vi "Save File Parse File Name RLT.vi"(8 "Error In":errorcluster, 11 "File String Name":path=path "C:/Users/220038920/Desktop/TR_S21_Lab ID_S21_SN_S21_Cycle_0_ClothWeight_8.45lbs_DOE_Exhaust_AHAM_20170703_File0_Inv and MC.csv") -> (0 "Error Out":errorcluster, 1 "Serial Number":string, 2 "Cycle":string, 3 "Date":string, 4 "Lab ID":string, 6 "TR Number":string)   [LabVIEW 2016, in "Save File.lvlib"]
uses:
  Save File.lvlib
  <vilib>/Utility/error.llb/whitespace.ctl
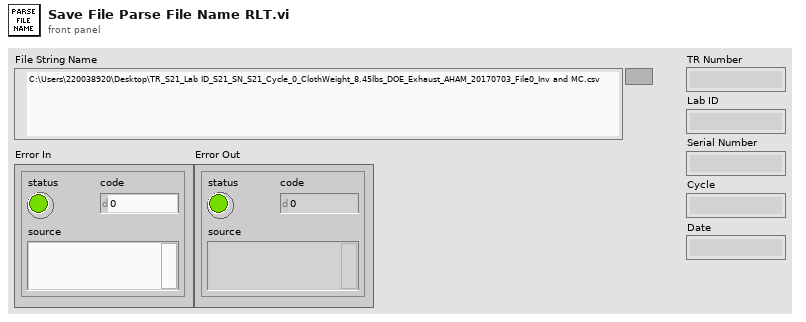
[diagram p1: front panel]
types:
  T1 = typedef "whitespace.ctl" = u16
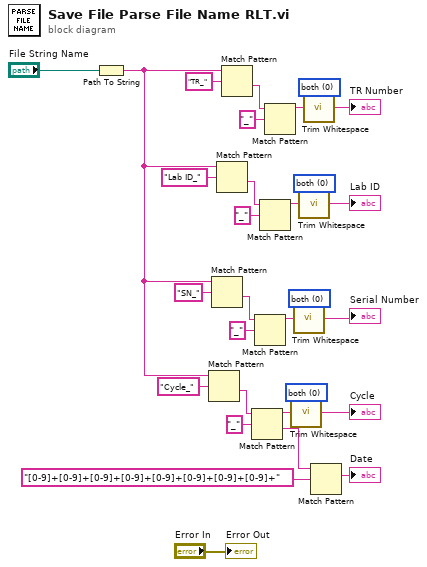
[diagram p0: block diagram]
diagram:
  w12 = T1 0 items=["both", "start of string", "end of string"] ("location (both)")
  w13 = T1 0 items=["both", "start of string", "end of string"] ("location (both)")
  w22 = T1 0 items=["both", "start of string", "end of string"] ("location (both)")
  w23 = T1 0 items=["both", "start of string", "end of string"] ("location (both)")
  n1 = Path To String(path="File String Name") -> (string=w4:string)
  n2 = Match Pattern(string=w4, regular expression="Cycle_") -> (after substring=w9:string)  [unwired: 1 in, 3 out]
  n3 = Match Pattern(string=w4, regular expression="SN_") -> (after substring=w16:string)  [unwired: 1 in, 3 out]
  n4 = Match Pattern(string=w4, regular expression="Lab ID_") -> (after substring=w19:string)  [unwired: 1 in, 3 out]
  n5 = Match Pattern(string=w4, regular expression="TR_") -> (after substring=w27:string)  [unwired: 1 in, 3 out]
  n6 = Match Pattern(string=w9, regular expression="_") -> (before substring=w11:string, after substring=w2:string)  [unwired: 1 in, 2 out]
  n7 = Match Pattern(string=w16, regular expression="_") -> (before substring=w14:string)  [unwired: 1 in, 3 out]
  n8 = Match Pattern(string=w19, regular expression="_") -> (before substring=w21:string)  [unwired: 1 in, 3 out]
  n9 = Match Pattern(string=w27, regular expression="_") -> (before substring=w25:string)  [unwired: 1 in, 3 out]
  n10 = call <vilib>:"Trim Whitespace.vi"("string"=w11, "location (both)"=w12) -> ("trimmed string"=→"Cycle":string)
  n11 = call <vilib>:"Trim Whitespace.vi"("string"=w14, "location (both)"=w13) -> ("trimmed string"=→"Serial Number":string)
  n12 = call <vilib>:"Trim Whitespace.vi"("string"=w21, "location (both)"=w22) -> ("trimmed string"=→"Lab ID":string)
  n13 = call <vilib>:"Trim Whitespace.vi"("string"=w25, "location (both)"=w23) -> ("trimmed string"=→"TR Number":string)
  n14 = Match Pattern(string=w2, regular expression="[0-9]+[0-9]+[0-9]+[0-9]+[0-9]+[0-9]+[0-9]+[0-9]+") -> (match substring=→"Date":string)  [unwired: 1 in, 3 out]
  "Error Out" <- "Error In"
